vi "Process Data.vi"(8 "error in (no error)":errorcluster, 10 "AbstractData in":refnum<class "AbstractData.lvclass">, 11 "AbstractProcessor2D in":refnum<class "AbstractProcessor2D.lvclass">) -> (0 "error out":errorcluster, 2 "AbstractData out":refnum<class "AbstractData.lvclass">, 3 "AbstractProcessor2D out":refnum<class "AbstractProcessor2D.lvclass">)   [LabVIEW 2014, in "AbstractProcessor2D.lvclass"]
uses:
  AbstractProcessor2D.lvclass
  Model/Data/AbstractData/AbstractData.lvclass
  Model/Data/Data2D/Data2D.lvclass
  Data2D Cluster.ctl
  Interfaces/Observable Actor/Observable Actor.lvclass
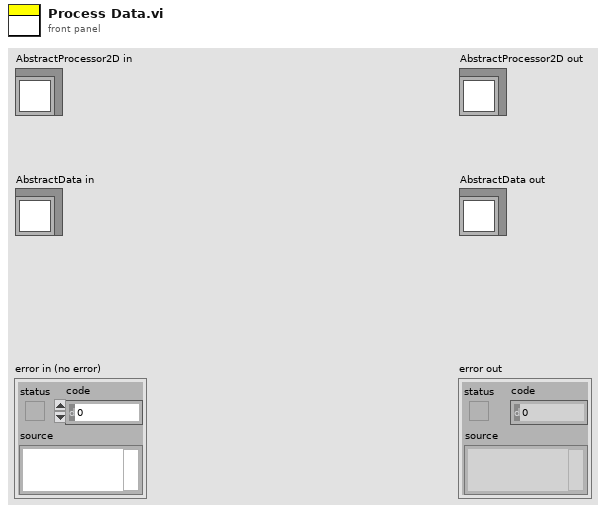
[diagram p1: front panel]
types:
  T1 = typedef "AbstractProcessor2D.lvclass/Data2D Cluster.ctl" = cluster{"in":refnum<class "Data2D.lvclass">, "out":refnum<class "Data2D.lvclass">}
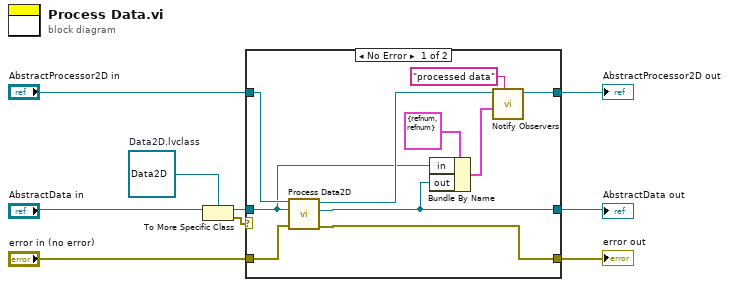
[diagram p0: block diagram]
diagram:
  w1 = refnum<class "Data2D.lvclass"> refnum  # Data2D.lvclass
  n1 = To More Specific Class(target class=w1, reference="AbstractData in") -> (specific class reference=w9:refnum<class "Data2D.lvclass">, error out=w8:errorcluster)  [unwired: 1 in]
  n2 = case shown="No Error" w8 {
    tunnel: w9 -> [w11 w20]
    tunnel: "error in (no error)" -> [w15 w22]
    tunnel: [w12 w22] -> w7
    tunnel: "AbstractProcessor2D in" -> [w16 w21]
    tunnel: [w18 w21] -> w3
    tunnel: [w13 w20] -> w2
    frame No Error {
      n3 = call-dynamic "Process Data2D.vi"("error in (no error)"=w15, "Data2D in"=w11, "AbstractProcessor2D in"=w16) -> ("error out"=w12:errorcluster, "Data2D out"=w13:refnum<class "Data2D.lvclass">, "AbstractProcessor2D out"=w14:refnum<class "AbstractProcessor2D.lvclass">)  [unwired: 6 in]
      n4 = Bundle By Name(cluster=T1 {"in"=refnum, "out"=refnum} ("Cluster"), "in"=w11, "out"=w13) -> (w19:T1)
      n5 = call "Notify Observers.vi"("name"="processed data", "value"=w19, "Observable Actor in"=w14) -> ("Observable Actor out"=w18:refnum<class "AbstractProcessor2D.lvclass">)  [unwired: 7 in, 1 out]
    }
    frame Error {
    }
  }
  "error out" <- w7
  "AbstractProcessor2D out" <- w3
  "AbstractData out" <- w2
